vi "Add Error.vi"(8 "error in (no error)":errorcluster, 10 "error code (0)":i32, 11 "error?":bool) -> (0 "error out":errorcluster)   [LabVIEW 2016]
doc: "If there is an error, add the following error code and its message to the error cluster. Error messages are taken from the configuration file in the section errors with the key equal to the error code."
uses:
  Get Key String.vi
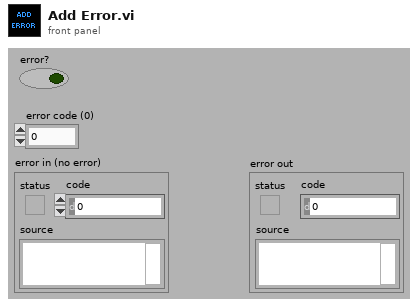
[diagram p1: front panel]
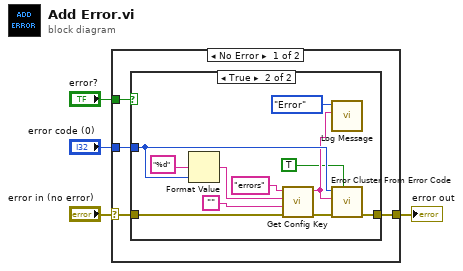
[diagram p0: block diagram]
diagram:
  n1 = case shown="No Error" "error in (no error)" {
    selector: "error in (no error)" -> [w6 w21]
    tunnel: "error code (0)" -> [w8 _]
    tunnel: [w7 w21] -> w3
    tunnel: "error?" -> [w5 _]
    frame No Error {
      n2 = case shown="True" w5 {
        tunnel: w8 -> [_ w16]
        tunnel: [w9 w14] -> w7
        tunnel: w6 -> [w9 w13]
        frame False {
        }
        frame True {
          n3 = Format Value(format string="%d", value (0)=w16) -> (output string=w19:string)  [unwired: 1 in]
          n4 = call-poly "Get Config Key.vi"("error in (no error)"=w13, "default value"="", "key"=w19, "section"="errors") -> ("error out"=w15:errorcluster, "value"=w11:string)  [unwired: 6 in]
          n5 = call "Log Message.vi"("message"=w11, "Type"=enum16{"Error", "Warning", "Note"}."Error") -> ()  [unwired: 9 in]
          n6 = call <vilib>:"Error Cluster From Error Code.vi"("show call chain? (False)"=TRUE, "error in (no error)"=w15, "error message (\"\")"=w11, "error code (0)"=w16) -> ("error out"=w14:errorcluster)  [unwired: 5 in]
        }
      }
    }
    frame Error {
    }
  }
  "error out" <- w3
